vi "Init.vi"(8 "error in (no error)":errorcluster, 9 "SubQueueIN":refnum<queue>, 10 "MainQueueIN":refnum<queue>, 11 "Data Value Reference IN":refnum<data-value>) -> (0 "error out":errorcluster, 3 "Data Value Reference out":refnum<data-value>)   [LabVIEW 2013]
uses:
  Control/SystemCommand.ctl
  Control/SystemData.ctl
  Control/SignalType.ctl
  Control/SubDaqCommand.ctl
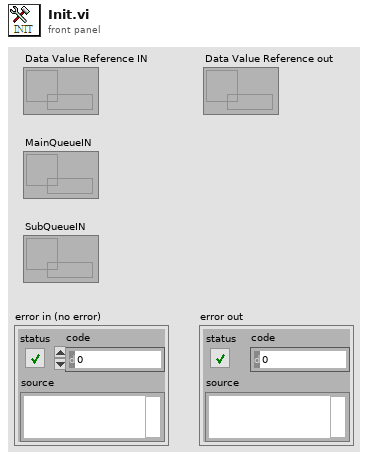
[diagram p1: front panel]
types:
  T1 = typedef "SystemCommand.ctl" = enum16{"None", "Init", "Close", "ShowNumeric", "ShowString", "ShowBool", "SquareNumeric", "ReverseString", "InvertBool", "FFT"}
  T2 = typedef "SystemData.ctl" = cluster{"Numeric":dbl, "String":string, "Boolean":bool, "Frequency":dbl, "Amplitude":dbl, "SignalType":T3, "WaveformArray":waveform(dbl)[], "Reset":bool, "StateString":string, "FFTmagnitudes":cluster{"f0":dbl, "df":dbl, "magnitude":dbl[]}[]}
  T3 = typedef "SignalType.ctl" = enum16{"Sin", "Triangle", "Square"}
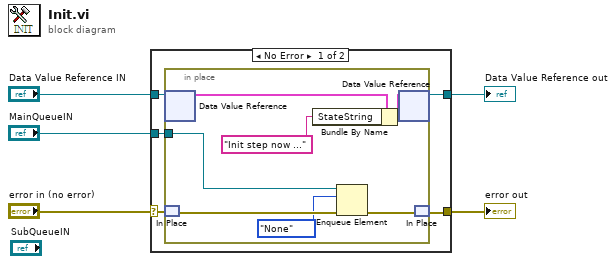
[diagram p0: block diagram]
diagram:
  n1 = case shown="No Error" "error in (no error)" {
    selector: "error in (no error)" -> [w10 w18]
    tunnel: "Data Value Reference IN" -> [w8 w19]
    tunnel: [w7 w19] -> w2
    tunnel: [w9 w18] -> w4
    tunnel: "MainQueueIN" -> [w6 _]
    frame No Error {
      n2 = in-place {
        in-place-border: w6 -> [w12]
        n3 = in-place-dvr #1(w8) -> (w17:T2)  [unwired: 1 out]
        n4 = in-place-match #2(w10) -> (w14:errorcluster)
        n5 = Bundle By Name(cluster=w17, "StateString"="Init step now ..." ("message")) -> (w16:T2)
        n6 = Enqueue Element(queue=w12, element=SystemCommand."None", error in (no error)=w14) -> (error out=w13:errorcluster)  [unwired: 1 in, 2 out]
        n7 = in-place-dvr #1(w16) -> (w7:refnum<data-value>)  [unwired: 1 out]
        n8 = in-place-match #2(w13) -> (w9:errorcluster)
      }
    }
    frame Error {
    }
  }
  "error out" <- w4
  "Data Value Reference out" <- w2
